vi "Write Sample.vi"(8 "error in (no error)":errorcluster, 10 "Sample.lvclass":refnum<class "Sample.lvclass">, 11 "Capillary Line in":refnum<class "Capillary Line.lvclass">) -> (0 "error out":errorcluster, 3 "Capillary Line out":refnum<class "Capillary Line.lvclass">)   [LabVIEW 2015, in "cRIO-Carbondioxide.lvlib" / "CO2-Actor.lvlib" / "Capillary Line.lvclass"]
uses:
  Capillary Line.lvclass
  subs/Sample/Sample.lvclass
  Capillary Line.lvclass/Capillary Line.ctl
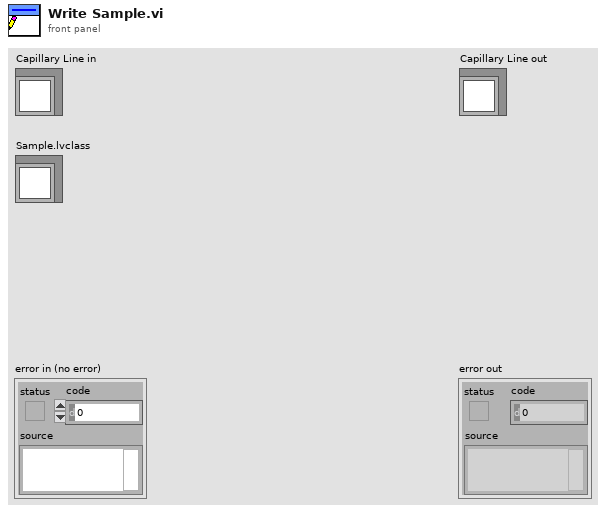
[diagram p1: front panel]
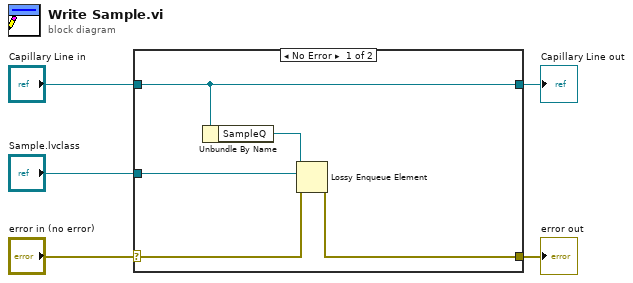
[diagram p0: block diagram]
diagram:
  n1 = case shown="No Error" "error in (no error)" {
    selector: "error in (no error)" -> [w8 w11]
    tunnel: [w7 w11] -> w4
    tunnel: [w6 w12] -> w2
    tunnel: "Capillary Line in" -> [w6 w12]
    tunnel: "Sample.lvclass" -> [w9 _]
    frame No Error {
      n2 = Unbundle By Name(w6) -> ("SampleQ"=w10:refnum<queue>)
      n3 = Lossy Enqueue Element(queue=w10, element=w9, error in (no error)=w8) -> (error out=w7:errorcluster)  [unwired: 3 out]
    }
    frame Error {
    }
  }
  "error out" <- w4
  "Capillary Line out" <- w2
